vi "Agilent N6900 N7900 Series Output DC Volts.vi"() -> ()   [LabVIEW 2021]
doc: "This example shows how to configure the instrument's output voltage level. The average voltage level and average current level are returned."
uses:
  <instrlib>/Agilent N6900 N7900 Series/Agilent N6900 N7900 Series.lvlib
panel:
  in  "Enable OCP (F: Disabled)":bool
  in  "OCP Delay Time Start Type (0: Command Changed)":u16(ring) items=["Command Changed", "Any Transition Method"]
  in  "OVP Protection (48V)":dbl=48.0
  in  "Voltage Priority Current Upper Limit (2.50A)":dbl=2.5
  in  "Voltage Priority Current Lower Limit (-2.50A)":dbl=-2.5
  in  "Voltage Immediate Amplitude (0 V)":dbl
  in  "Stop Output":bool
  out "Average Current Level (A)":dbl format="%.2f"
  out "Average Voltage Level (V)":dbl format="%.2f"
  in  "VISA resource name":refnum<visa-resource-name>
  # "(c) 2013-2018 National Instruments Corporation.  ALL RIGHTS RESERVED."
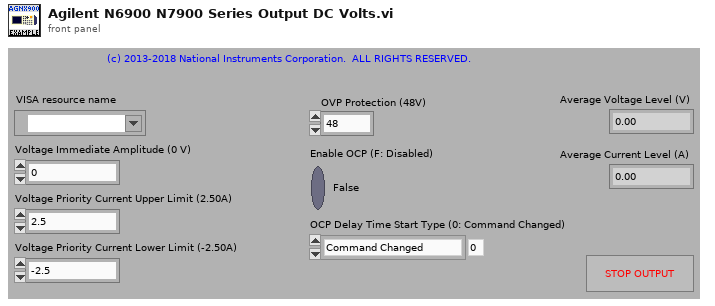
[diagram p1: front panel]
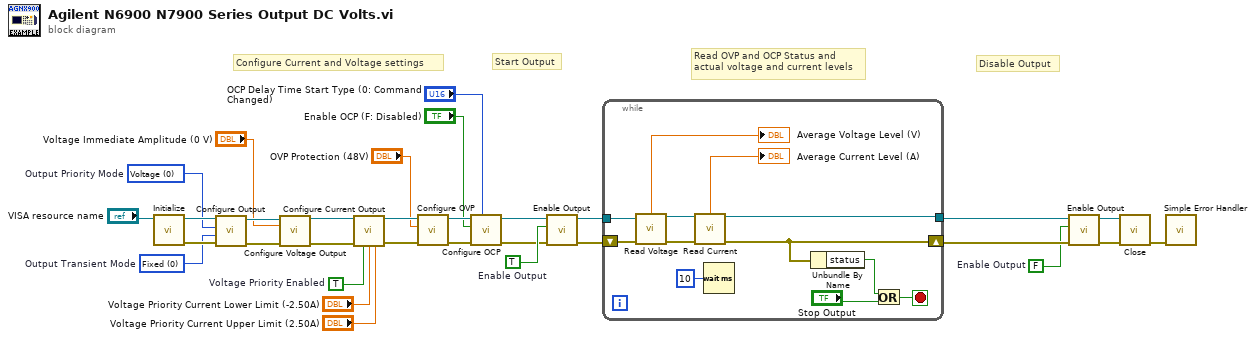
[diagram p0: block diagram]
diagram:
  w10 = FALSE  # Enable Output
  w23 = TRUE  # Enable Output
  w13 = TRUE  # Voltage Priority Enabled
  w26 = u16 0 items=["Fixed", "Step", "List", "Arbitrary"]  # Output Transient Mode
  w27 = u16 0 items=["Voltage", "Current"]  # Output Priority Mode
  # "Configure Current and Voltage settings"
  # "Disable Output"
  # "Read OVP and OCP Status and\nactual voltage and current levels"
  # "Start Output"
  n1 = call <instrlib>:"Initialize.vi"("VISA resource name"="VISA resource name") -> ("error out"=w28:errorcluster, "VISA resource name out"=w29:refnum<visa-resource-name>)  [unwired: 9 in]
  n2 = call <instrlib>:"Configure Output.vi"("error in (no error)"=w28, "Output Transient Mode (0: Fixed)"=w26, "Output Priority Mode (0: Voltage)"=w27, "VISA resource name"=w29) -> ("error out"=w17:errorcluster, "VISA resource name out"=w18:refnum<visa-resource-name>)  [unwired: 6 in]
  n3 = call <instrlib>:"Configure Voltage Output.vi"("VISA resource name"=w18, "Voltage Immediate Amplitude (0 V)"="Voltage Immediate Amplitude (0 V)", "error in (no error)"=w17) -> ("VISA resource name out"=w15:refnum<visa-resource-name>, "error out"=w14:errorcluster)  [unwired: 11 in]
  n4 = call <instrlib>:"Configure Current Output.vi"("VISA resource name"=w15, "error in (no error)"=w14, "Enable Voltage Priority (False)"=w13, "Voltage Priority Current Lower Limit (-2.50A)"="Voltage Priority Current Lower Limit (-2.50A)", "Voltage Priority Current Upper Limit (2.50A)"="Voltage Priority Current Upper Limit (2.50A)") -> ("VISA resource name out"=w9:refnum<visa-resource-name>, "error out"=w8:errorcluster)  [unwired: 9 in]
  n5 = call <instrlib>:"Configure OVP.vi"("error in (no error)"=w8, "OVP Protection (48V)"="OVP Protection (48V)", "VISA resource name"=w9) -> ("error out"=w5:errorcluster, "VISA resource name out"=w6:refnum<visa-resource-name>)  [unwired: 7 in]
  n6 = call <instrlib>:"Configure OCP.vi"("OCP Delay Time Start Type (0: Command Changed)"="OCP Delay Time Start Type (0: Command Changed)", "error in (no error)"=w5, "Enable OCP (F: Disabled)"="Enable OCP (F: Disabled)", "VISA resource name"=w6) -> ("error out"=w4:errorcluster, "VISA resource name out"=w3:refnum<visa-resource-name>)  [unwired: 6 in]
  n7 = call <instrlib>:"Enable Output.vi"("error in (no error)"=w4, "Enable Output (F: Disable)"=w23, "VISA resource name"=w3) -> ("error out"=w24:errorcluster, "VISA resource name out"=w25:refnum<visa-resource-name>)  [unwired: 7 in]
  n8 = while {
    tunnel: [w34] -> w19
    shift-right: [w33] -> w20
    shift-left: w24 -> [w39]
    tunnel: w25 -> [w40]
    stop <- w43 stop-if-true
    n9 = call <instrlib>:"Read Voltage.vi"("VISA resource name"=w40, "error in (no error)"=w39) -> ("Average Voltage"=→"Average Voltage Level (V)":dbl, "VISA resource name out"=w37:refnum<visa-resource-name>, "error out"=w36:errorcluster)  [unwired: 6 in, 5 out]
    n10 = call <instrlib>:"Read Current.vi"("VISA resource name"=w37, "error in (no error)"=w36) -> ("Average Current"=→"Average Current Level (A)":dbl, "VISA resource name out"=w34:refnum<visa-resource-name>, "error out"=w33:errorcluster)  [unwired: 6 in, 5 out]
    n11 = Wait (ms)(milliseconds to wait=u32 10) -> ()  [unwired: 1 out]
    n12 = Unbundle By Name(w33) -> ("status"=w41:bool)
    n13 = Or(x=w41, y="Stop Output") -> (x .or. y?=w43:bool)
  }
  n14 = call <instrlib>:"Enable Output.vi"("error in (no error)"=w20, "Enable Output (F: Disable)"=w10, "VISA resource name"=w19) -> ("error out"=w22:errorcluster, "VISA resource name out"=w21:refnum<visa-resource-name>)  [unwired: 7 in]
  n15 = call <instrlib>:"Close.vi"("error in (no error)"=w22, "VISA resource name"=w21) -> ("error out"=w30:errorcluster)  [unwired: 9 in]
  n16 = call <vilib>:"Simple Error Handler.vi"("error in (no error)"=w30) -> ()  [unwired: 4 in, 5 out]
